vi "Server.vi"   [LabVIEW 2025]
uses:
  ServerGlobalVariables.vi
  ServerNetworkInterfaceGlobalVariables.vi
  <vilib>/Utility/miscctls.llb/LVMapReplaceAction.ctl
  bb7a831f-7d97-4d2b-be74-8b4a38f97bb1.vi
types:
  T1 = map{u32, cluster{"Name":string, "Team":u8, "Ready":bool, "Host":bool, "Alive":bool, "Color":u32, "Lands":set{cluster{"Row":u32, "Column":u32}}, "Army":u32}}
  T2 = enum16{"Init", "Lobby", "Game Init", "Game", "Game End"}
  T3 = enum16{"Wait Send Queue Ready", "Wait Receive Queue Ready", "Poll Read Queue", "Process Data"}
  T4 = cluster{"Data":string, "Address":u32, "Port":u16}
  T5 = enum16{"Wait Send Queue Ready", "Wait Receive Queue Ready", "Poll Read Queue", "Process Data", "Remove Land"}
  T6 = typedef "LVMapReplaceAction.ctl" = enum32{"Modify Entry only if found", "Add or Modify Entry", "Delete Entry"}
  T7 = cluster{"Name":string, "Team":u8, "Ready":bool, "Host":bool, "Alive":bool, "Color":u32, "Lands":set{cluster{"Row":u32, "Column":u32}}, "Army":u32}
  T8 = cluster{"string array[0]":string, "string array[1]":string, "string array[2]":string, "string array[3]":string}
  T9 = cluster{"Troops":u32, "Owner":i32, "Mountain":bool, "City":bool, "General":bool}[][]
  T10 = cluster{"Troops":u32, "Owner":i32, "Mountain":bool, "City":bool, "General":bool}
  T11 = cluster{"string array[0]":string, "string array[1]":string}
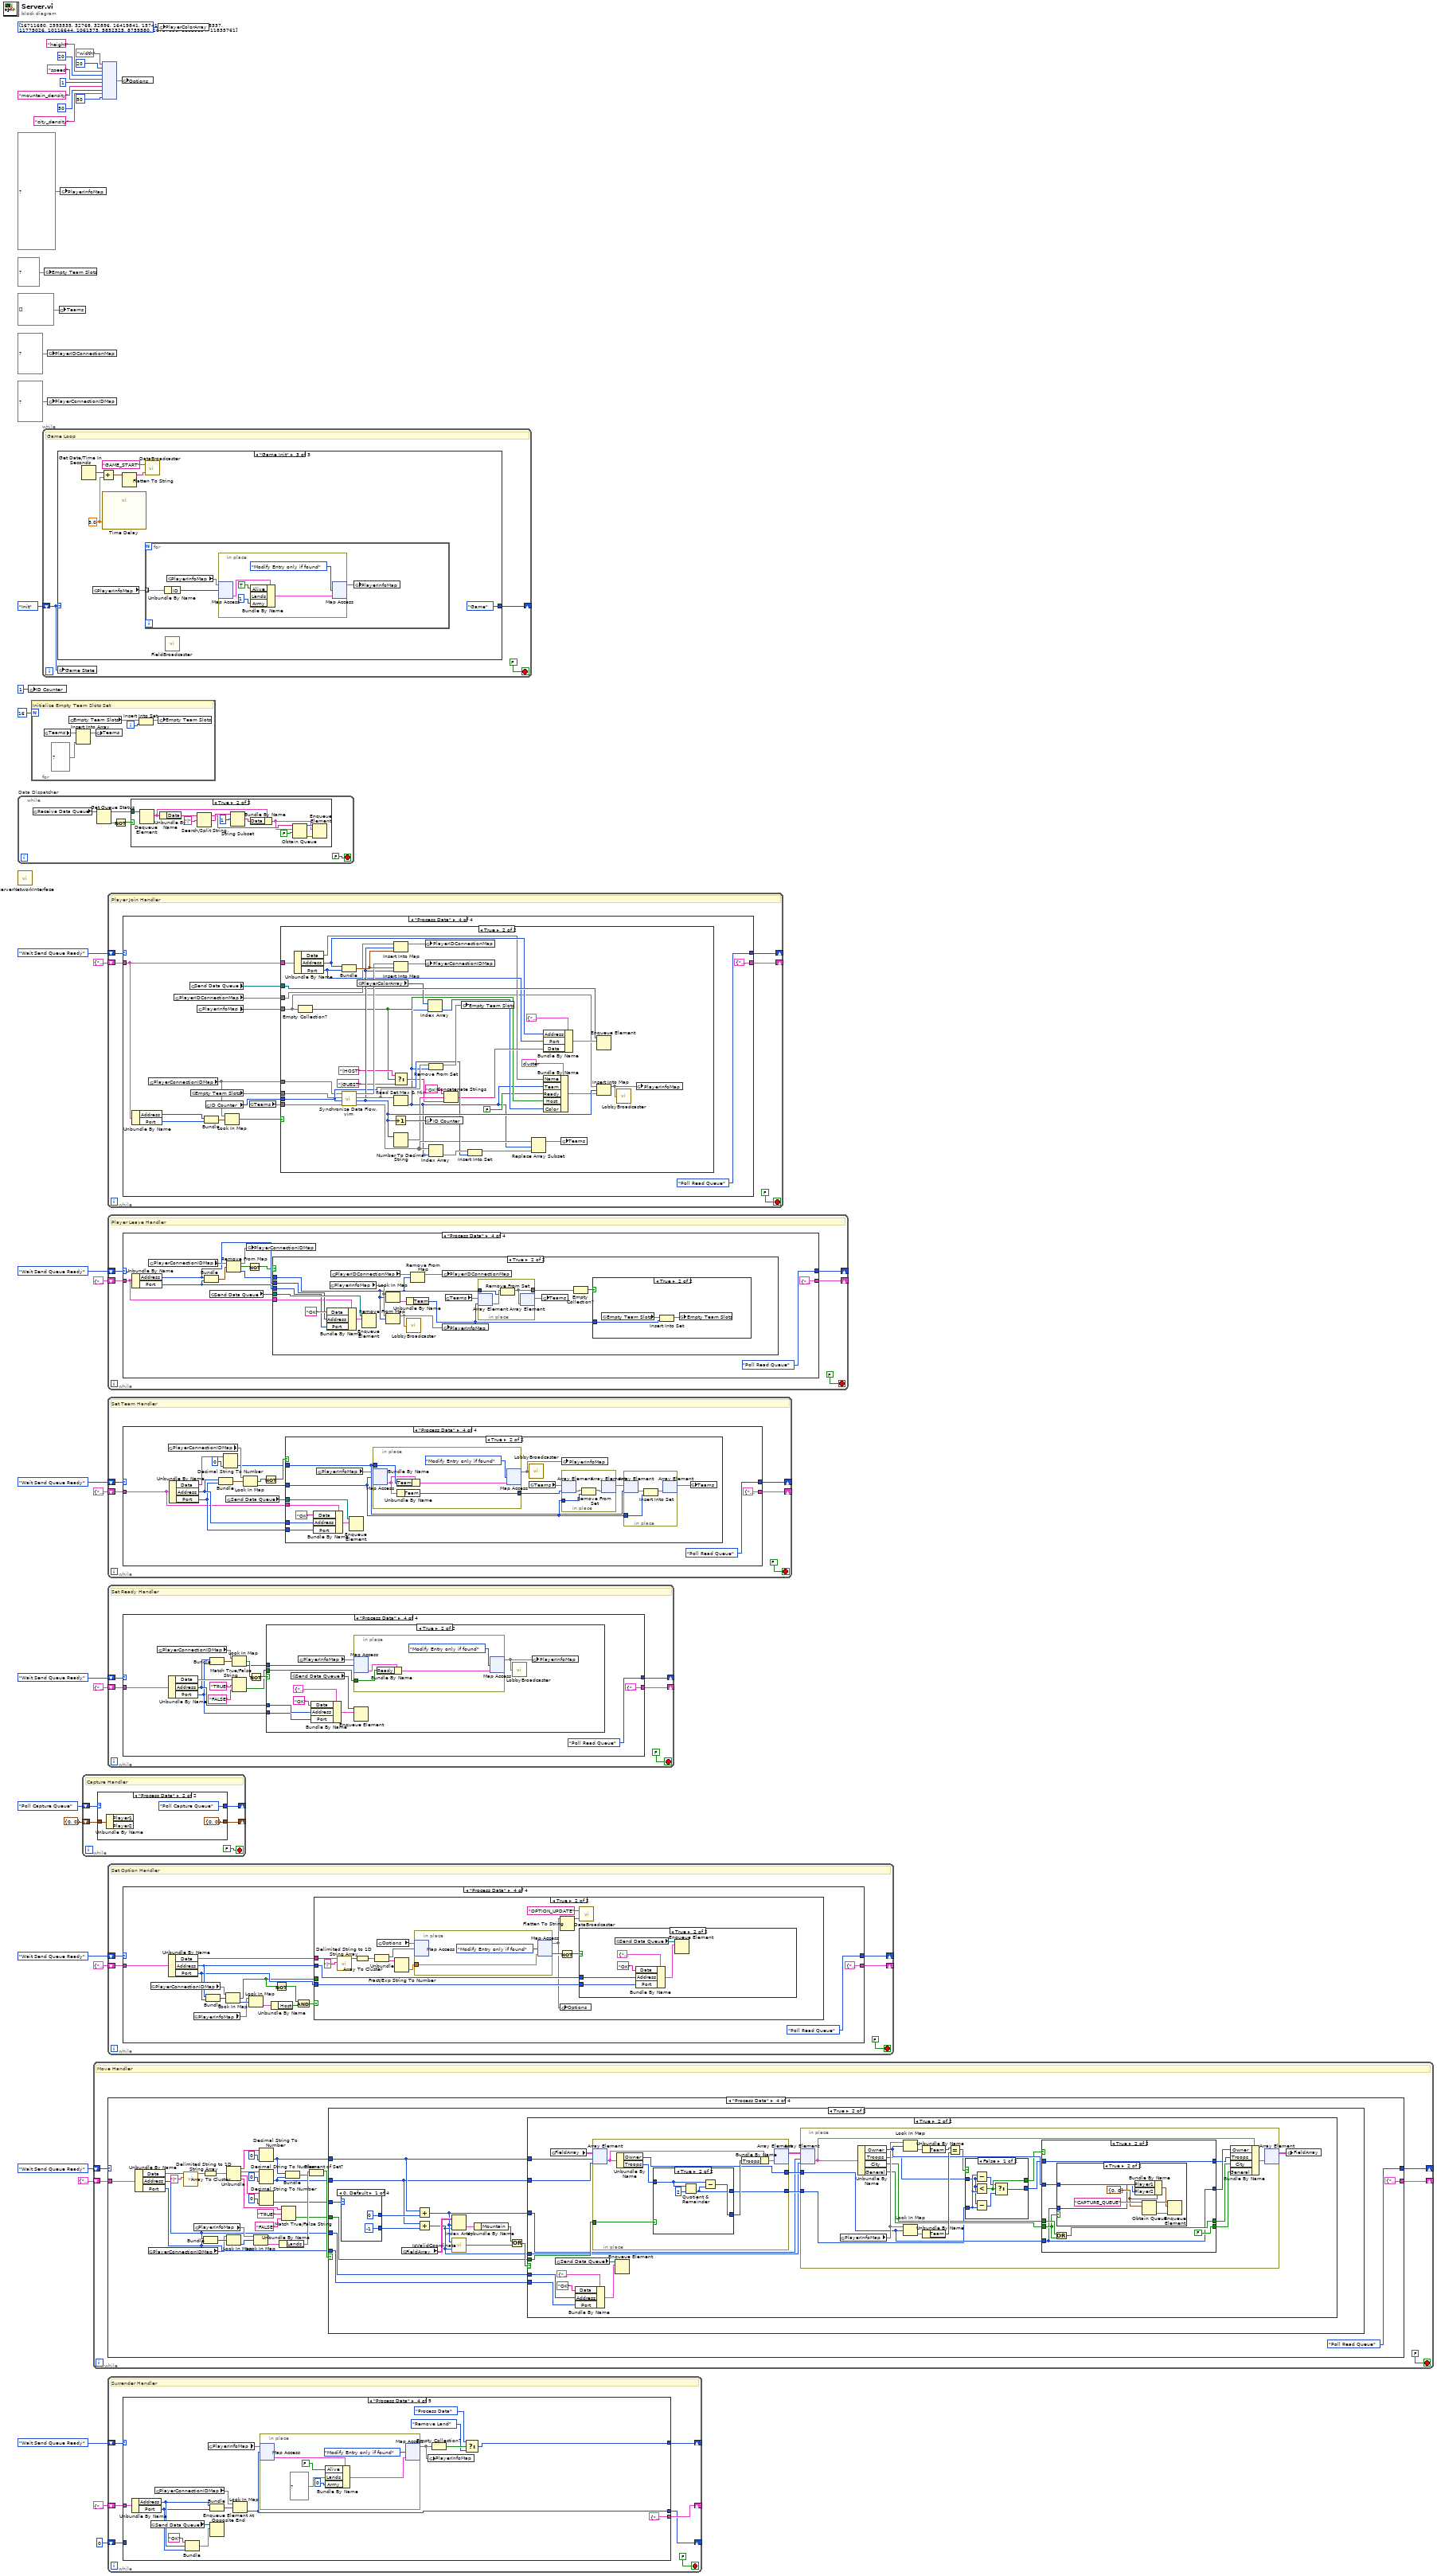
[diagram p0: block diagram]
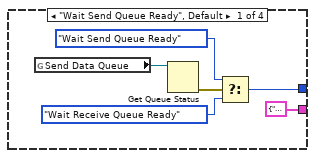
[diagram p2: hidden frame]
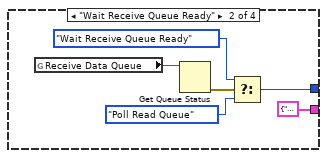
[diagram p3: hidden frame]
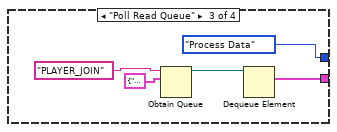
[diagram p4: hidden frame]
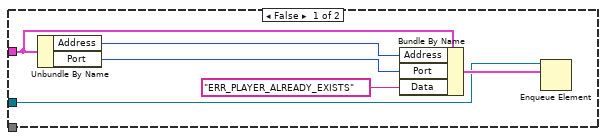
[diagram p5: hidden frame]
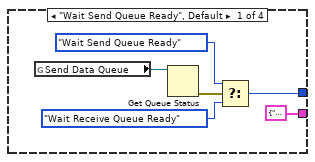
[diagram p6: hidden frame]
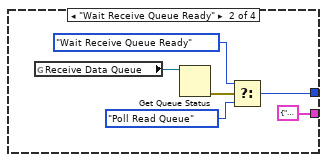
[diagram p7: hidden frame]
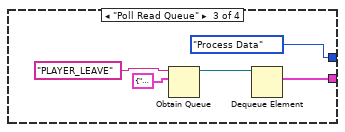
[diagram p8: hidden frame]
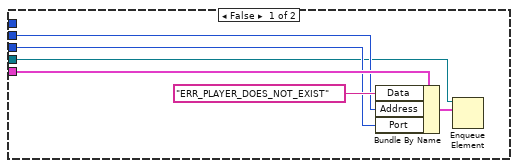
[diagram p9: hidden frame]
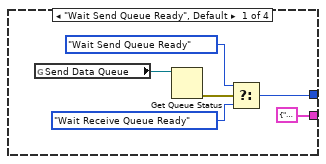
[diagram p11: hidden frame]
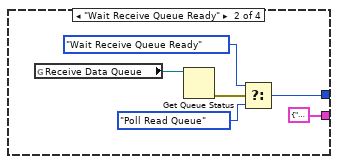
[diagram p12: hidden frame]
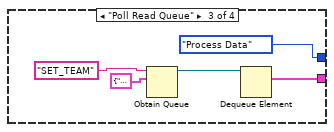
[diagram p13: hidden frame]
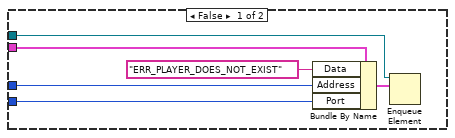
[diagram p14: hidden frame]
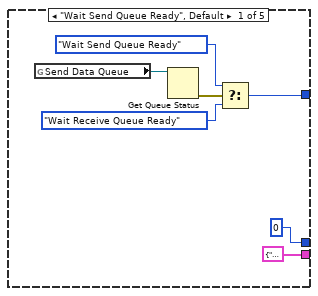
[diagram p15: hidden frame]
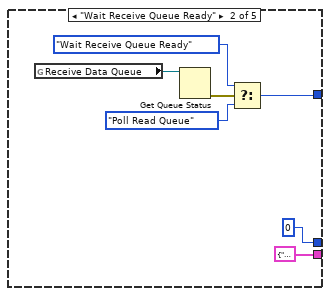
[diagram p16: hidden frame]
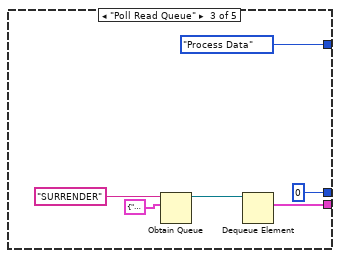
[diagram p17: hidden frame]
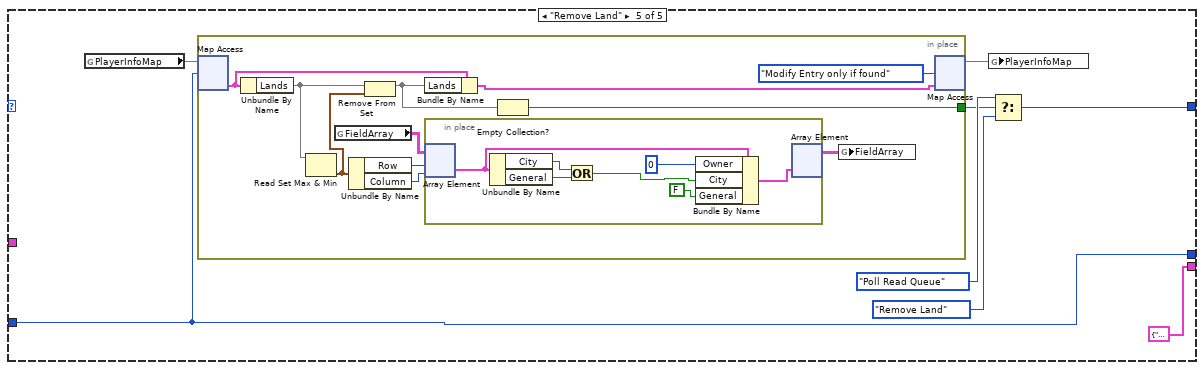
[diagram p18: hidden frame]
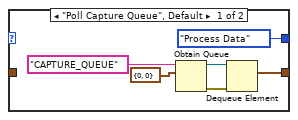
[diagram p19: hidden frame]
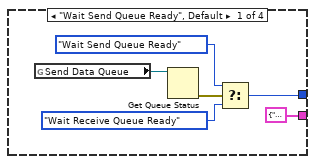
[diagram p20: hidden frame]
diagram:
  n1 = while "Data Dispatcher" {
    stop <- FALSE stop-if-true
    n2 = global read "ServerNetworkInterfaceGlobalVariables.vi" "Receive Data Queue"() -> (w41:refnum<queue>)
    n3 = Get Queue Status(queue=w41) -> (queue out=w38:refnum<queue>, error out=w40:errorcluster)  [unwired: 2 in, 6 out]
    n4 = Not(x=w40) -> (.not. x?=w39:bool)
    n5 = case shown="True" w39 {
      tunnel: w38 -> [_ w43]
      frame False {
      }
      frame True {
        n6 = Dequeue Element(queue=w43) -> (element=w50:T4)  [unwired: 2 in, 3 out]
        n7 = Unbundle By Name(w50) -> ("Data"=w54:string)
        n8 = Search/Split String(string=w54, search string/char (-)="|") -> (substring before match=w47:string, match + rest of string=w52:string)  [unwired: 1 in, 1 out]
        n9 = String Subset(string=w52, offset (0)=1) -> (substring=w49:string)  [unwired: 1 in]
        n10 = Bundle By Name(cluster=w50, "Data"=w49) -> (w44:T4)
        n11 = Obtain Queue(name (unnamed)=w47, element data type=w44, create if not found? (T)=FALSE) -> (queue out=w46:refnum<queue>, error out=w45:errorcluster)  [unwired: 2 in, 1 out]
        n12 = Enqueue Element(queue=w46, element=w44, error in (no error)=w45) -> ()  [unwired: 1 in, 3 out]
      }
    }
  }
  n13 = call "ServerNetworkInterface.vi"() -> ()  [unwired: 1 in]
  n14 = global write "ServerGlobalVariables.vi" "ID Counter"(u32 1 ("ID Counter")) -> ()
  n15 = for {
    N: 16 -> [_]
    i -> [w55]
    # "Initialize Empty Team Slots Set"
    n16 = global read "ServerGlobalVariables.vi" "Teams"() -> (w57:set{u32}[])
    n17 = global read "ServerGlobalVariables.vi" "Empty Team Slots"() -> (w60:set{u8})
    n18 = Insert Into Array(array=w57, new element=set{u32} {} ("new element/subarray")) -> (w58:set{u32}[])  [unwired: 1 in]
    n19 = global write "ServerGlobalVariables.vi" "Teams"(w58) -> ()
    n20 = Insert Into Set(10:w55, 11:w60) -> (3:w59:set{u8})  [unwired: 1 out]
    n21 = global write "ServerGlobalVariables.vi" "Empty Team Slots"(w59) -> ()
  }
  n22 = while {
    shift-right: [w61] -> _
    shift-left: T2."Init" -> [w62]
    stop <- FALSE stop-if-true
    # "Game Loop"
    n23 = case shown="\"Game Init\"" w62 {
      tunnel: [T2."Init" w65 T2."Game"] -> w61
      frame "Init", Default {
      }
      frame "Lobby" {
        n24 = global read "ServerGlobalVariables.vi" "PlayerInfoMap"() -> (w69:T1)
        n25 = Collection Size(1:w69) -> (0:w71:i32)
        n26 = for {
          N: w71 -> [_]
          shift-right: [w74] -> w68
          shift-left: TRUE -> [w72]
          tunnel: w69 -> [w75] mode=indexing
          n27 = Unbundle By Name(w75) -> ("PlayerInfo.Ready"=w73:bool)
          n28 = And(x=w73, y=w72) -> (x .and. y?=w74:bool)
        }
        n29 = Select(t=T2."Lobby", s=w68, f=T2."Game Init") -> (s? t:f=w65:T2)
      }
      frame "Game Init" {
        w77 = 3.0 ("y")
        n30 = Get Date/Time In Seconds() -> (seconds since 1Jan1904=w80:timestamp)
        n31 = global read "ServerGlobalVariables.vi" "PlayerInfoMap"() -> (w76:T1)
        n32 = Add(x=w80, y=w77) -> (x+y=w78:timestamp)
        n33 = call "Time Delay"("Delay Time (s)"=w77) -> ()  [unwired: 10 in, 1 out]
        n34 = Flatten To String(anything=w78) -> (data string=w79:string)  [unwired: 3 in, 2 out]
        n35 = call "DataBroadcaster.vi"("Data"=w79, "Action"="GAME_START") -> ()
        n36 = for {
          tunnel: w76 -> [w86] mode=indexing
          n37 = Unbundle By Name(w86) -> ("ID"=w84:u32)
          n38 = global read "ServerGlobalVariables.vi" "PlayerInfoMap"() -> (w85:T1)
          n39 = in-place {
            n40 = in-place-map #1(w85, w84) -> (w91:T7)  [unwired: 1 in, 1 out]
            n41 = Bundle By Name(cluster=w91, "Alive"=TRUE, "Army"=u32 1) -> (w88:T7)  [unwired: 1 in]
            n42 = in-place-map #1(w88, LVMapReplaceAction."Modify Entry only if found" ("action")) -> (w83:T1)  [unwired: 2 out]
          }
          n43 = global write "ServerGlobalVariables.vi" "PlayerInfoMap"(w83) -> ()
        }
        n44 = call "FieldBroadcaster.vi"() -> ()  [unwired: 12 in]
      }
    }
    n45 = global write "ServerGlobalVariables.vi" "Game State"(w62) -> ()
  }
  n46 = global write "ServerGlobalVariables.vi" "Empty Team Slots"(set{u8} {} ("Empty Team Slots")) -> ()
  n47 = global write "ServerGlobalVariables.vi" "PlayerIDConnectionMap"(map{u32, cluster{"Address":u32, "Port":u16}} {} ("PlayerIDConnectionMap")) -> ()
  n48 = global write "ServerGlobalVariables.vi" "PlayerConnectionIDMap"(map{cluster{"Address":u32, "Port":u16}, u32} {} ("PlayerConnectionIDMap")) -> ()
  n49 = global write "ServerGlobalVariables.vi" "Teams"(set{u32}[] [] ("Teams")) -> ()
  n50 = global write "ServerGlobalVariables.vi" "PlayerInfoMap"(T1 {} ("PlayerInfoMap")) -> ()
  n51 = while {
    shift-right: [w95] -> _
    shift-left: enum16{"Poll Capture Queue", "Process Data"}."Poll Capture Queue" -> [w96]
    shift-right: [w94] -> _
    shift-left: cluster{"Player1":u8, "Player2":u8} {"Player1"=0, "Player2"=0} -> [w93]
    stop <- FALSE stop-if-true
    # "Capture Handler"
    n52 = case shown="\"Process Data\"" w96 {
      tunnel: [enum16{"Poll Capture Queue", "Process Data"}."Process Data" enum16{"Poll Capture Queue", "Process Data"}."Poll Capture Queue"] -> w95
      tunnel: [w97 cluster{"Player1":u8, "Player2":u8} {"Player1"=0, "Player2"=0}] -> w94
      tunnel: w93 -> [_ w103]
      frame "Poll Capture Queue", Default {
        n53 = Obtain Queue(name (unnamed)="CAPTURE_QUEUE", element data type=cluster{"Player1":u8, "Player2":u8} {"Player1"=0, "Player2"=0}) -> (queue out=w99:refnum<queue>, error out=w98:errorcluster)  [unwired: 3 in, 1 out]
        n54 = Dequeue Element(queue=w99, error in (no error)=w98) -> (element=w97:cluster{"Player1":u8, "Player2":u8})  [unwired: 1 in, 3 out]
      }
      frame "Process Data" {
        n55 = Unbundle By Name(w103) -> ()  [unwired: 2 out]
      }
    }
  }
  n56 = while {
    shift-right: [w109] -> _
    shift-left: T3."Wait Send Queue Ready" -> [w106]
    shift-right: [w108] -> _
    shift-left: T4 {"Data"="", "Address"=0, "Port"=0} -> [w107]
    stop <- FALSE stop-if-true
    # "Move Handler"
    n57 = case shown="\"Process Data\"" w106 {
      tunnel: [w114 w118 T3."Process Data" T3."Poll Read Queue"] -> w109
      tunnel: [T4 {"Data"="", "Address"=0, "Port"=0} T4 {"Data"="", "Address"=0, "Port"=0} w124 T4 {"Data"="", "Address"=0, "Port"=0}] -> w108
      tunnel: w107 -> [_ _ _ w137]
      frame "Wait Send Queue Ready", Default {
        n58 = global read "ServerNetworkInterfaceGlobalVariables.vi" "Send Data Queue"() -> (w116:refnum<queue>)
        n59 = Get Queue Status(queue=w116) -> (error out=w115:errorcluster)  [unwired: 2 in, 7 out]
        n60 = Select(t=T3."Wait Send Queue Ready", s=w115, f=T3."Wait Receive Queue Ready") -> (s? t:f=w114:T3)
      }
      frame "Wait Receive Queue Ready" {
        n61 = global read "ServerNetworkInterfaceGlobalVariables.vi" "Receive Data Queue"() -> (w121:refnum<queue>)
        n62 = Get Queue Status(queue=w121) -> (error out=w122:errorcluster)  [unwired: 2 in, 7 out]
        n63 = Select(t=T3."Wait Receive Queue Ready", s=w122, f=T3."Poll Read Queue") -> (s? t:f=w118:T3)
      }
      frame "Poll Read Queue" {
        n64 = Obtain Queue(name (unnamed)="MOVE", element data type=T4 {"Data"="", "Address"=0, "Port"=0}) -> (queue out=w125:refnum<queue>)  [unwired: 3 in, 2 out]
        n65 = Dequeue Element(queue=w125) -> (element=w124:T4)  [unwired: 2 in, 3 out]
      }
      frame "Process Data" {
        n66 = Unbundle By Name(w137) -> ("Data"=w148:string, "Address"=w132:u32, "Port"=w133:u16)
        n67 = global read "ServerGlobalVariables.vi" "PlayerConnectionIDMap"() -> (w154:map{cluster{"Address":u32, "Port":u16}, u32})
        n68 = call <vilib>:"Delimited String to 1D String Array.vi"("delimiter"="|", "delimited string"=w148) -> ("string array"=w149:string[])  [unwired: 9 in]
        n69 = global read "ServerGlobalVariables.vi" "PlayerInfoMap"() -> (w152:T1)
        n70 = Array To Cluster(array=w149) -> (cluster=w142:T8)
        n71 = Bundle("Address"=w132, "Port"=w133) -> (w155:cluster{"Address":u32, "Port":u16})  [unwired: 1 in]
        n72 = Unbundle(w142) -> ("string array[0]"=w138:string, "string array[1]"=w139:string, "string array[2]"=w140:string, "string array[3]"=w141:string)
        n73 = Look In Map(map=w154, key=w155) -> (value=w153:u32)  [unwired: 1 in, 1 out]
        n74 = Look In Map(map=w152, key=w153) -> (value=w151:T7)  [unwired: 1 in, 1 out]
        n75 = Decimal String To Number(string=w138, default (0L)=u32 0 ("default (0 I32)")) -> (number=w130:u32)  [unwired: 1 in, 1 out]
        n76 = Decimal String To Number(string=w139, default (0L)=u32 0 ("default (0 I32)")) -> (number=w129:u32)  [unwired: 1 in, 1 out]
        n77 = Decimal String To Number(string=w140, default (0L)=u32 0 ("default (0 I32)")) -> (number=w131:u32)  [unwired: 1 in, 1 out]
        n78 = Unbundle By Name(w151) -> ("Lands"=w136:set{cluster{"Row":u32, "Column":u32}})
        n79 = Match True/False String(2:"FALSE" ("false string"), 3:"TRUE" ("true string"), 4:w141) -> (0:w128:bool)  [unwired: 1 out]
        n80 = Bundle(w130, w129) -> (w135:cluster{u32, u32})  [unwired: 1 in]
        n81 = Element of Set?(10:w135, 11:w136) -> (3:w134:bool)
        n82 = case shown="True" w134 {
          tunnel: w133 -> [w159 w174]
          tunnel: w132 -> [w158 w175]
          tunnel: w131 -> [_ w178]
          tunnel: w130 -> [_ w167]
          tunnel: w129 -> [_ w166]
          tunnel: w128 -> [_ w168]
          frame False {
            n83 = global read "ServerNetworkInterfaceGlobalVariables.vi" "Send Data Queue"() -> (w160:refnum<queue>)
            n84 = Bundle By Name(cluster=T4 {"Data"="", "Address"=0, "Port"=0}, "Data"="ERR_NOT_OWN_LAND", "Address"=w158, "Port"=w159) -> (w162:T4)
            n85 = Enqueue Element(queue=w160, element=w162) -> ()  [unwired: 2 in, 3 out]
          }
          frame True {
            n86 = case shown="0, Default" w178 {
              tunnel: [-1 0 1 0] -> w177
              tunnel: [0 1 0 -1] -> w176
              frame 0, Default {
              }
              frame 1 {
              }
              frame 2 {
              }
              frame 3 {
              }
            }
            n87 = global read "ServerGlobalVariables.vi" "FieldArray"() -> (w173:T9)
            n88 = Add(x=w167, y=w176) -> (x+y=w165:u32)
            n89 = Add(x=w166, y=w177) -> (x+y=w164:u32)
            n90 = Index Array(array=w173, index (row)=w165, index (col)=w164) -> (element=w169:T10)
            n91 = call "IsValidCoordinate.vi"("Column"=w164, "Row"=w165) -> ("Valid"=w171:bool)
            n92 = Unbundle By Name(w169) -> ("Mountain"=w172:bool)
            n93 = Or(x=w172, y=w171) -> (x .or. y?=w170:bool)
            n94 = case shown="True" w170 {
              tunnel: w175 -> [w180 w192]
              tunnel: w174 -> [w179 w191]
              tunnel: w168 -> [_ w197]
              tunnel: w167 -> [_ w200]
              tunnel: w166 -> [_ w199]
              tunnel: w165 -> [_ w187]
              tunnel: w164 -> [_ w186]
              frame False {
                n95 = global read "ServerNetworkInterfaceGlobalVariables.vi" "Send Data Queue"() -> (w181:refnum<queue>)
                n96 = Bundle By Name(cluster=T4 {"Data"="", "Address"=0, "Port"=0}, "Data"="ERR_INVALID_MOVE", "Address"=w180, "Port"=w179) -> (w183:T4)
                n97 = Enqueue Element(queue=w181, element=w183) -> ()  [unwired: 2 in, 3 out]
              }
              frame True {
                n98 = global read "ServerGlobalVariables.vi" "FieldArray"() -> (w198:T9)
                n99 = global read "ServerNetworkInterfaceGlobalVariables.vi" "Send Data Queue"() -> (w193:refnum<queue>)
                n100 = Bundle By Name(cluster=T4 {"Data"="", "Address"=0, "Port"=0}, "Data"="OK", "Address"=w192, "Port"=w191) -> (w195:T4)
                n101 = in-place {
                  in-place-border: w197 -> [w251]
                  in-place-border: [w253] -> w190
                  in-place-border: [w252] -> w189
                  n102 = in-place-array #2(w198, w200, w199) -> (w256:T10)
                  n103 = Unbundle By Name(w256) -> ("Owner"=w253:i32, "Troops"=w257:u32)
                  n104 = case shown="True" w251 {
                    tunnel: [w264 w269] -> w254
                    tunnel: [w265 w267] -> w252
                    tunnel: w257 -> [w261 w266]
                    frame False {
                      n105 = Decrement(x=w261) -> (x-1=w262:u32)
                      n106 = Greater Than 0?(x=w261) -> (x > 0?=w263:bool)
                      n107 = Select(t=w262, s=w263, f=u32 0) -> (s? t:f=w265:u32)
                      n108 = Select(t=u32 1, s=w263, f=u32 0) -> (s? t:f=w264:u32)
                    }
                    frame True {
                      n109 = Quotient & Remainder(x=w266, y=u32 2) -> (floor(x/y)=w267:u32)  [unwired: 1 out]
                      n110 = Subtract(x=w266, y=w267) -> (x-y=w269:u32)
                    }
                  }
                  n111 = Bundle By Name(cluster=w256, "Troops"=w254) -> (w255:T10)
                  n112 = in-place-array #2(w255) -> (w188:T9)  [unwired: 2 out]
                }
                n113 = Enqueue Element(queue=w193, element=w195) -> ()  [unwired: 2 in, 3 out]
                n114 = in-place {
                  in-place-border: w190 -> [w204]
                  in-place-border: w189 -> [w203]
                  n115 = in-place-array #3(w188, w187, w186) -> (w202:T10)
                  n116 = global read "ServerGlobalVariables.vi" "PlayerInfoMap"() -> (w215:T1)
                  n117 = Unbundle By Name(w202) -> ("Owner"=w216:i32, "Troops"=w206:u32, "City"=w208:bool, "General"=w212:bool)
                  n118 = Look In Map(map=w215, key=w216) -> (value=w218:T7)  [unwired: 1 in, 1 out]
                  n119 = Look In Map(map=w215, key=w204) -> (value=w217:T7)  [unwired: 1 in, 1 out]
                  n120 = Unbundle By Name(w218) -> ("Team"=w219:u8)
                  n121 = Unbundle By Name(w217) -> ("Team"=w220:u8)
                  n122 = Equal?(x=w219, y=w220) -> (x = y?=w205:bool)
                  n123 = case shown="False" w205 {
                    tunnel: w206 -> [w242 w250]
                    tunnel: w203 -> [w243 w249]
                    tunnel: [w246 w248] -> w209
                    tunnel: [w244 FALSE] -> w207
                    frame False {
                      n124 = Subtract(x=w243, y=w242) -> (x-y=w241:u32)
                      n125 = Less?(x=w242, y=w243) -> (x < y?=w244:bool)
                      n126 = Subtract(x=w242, y=w243) -> (x-y=w245:u32)
                      n127 = Select(t=w241, s=w244, f=w245) -> (s? t:f=w246:u32)
                    }
                    frame True {
                      n128 = Add(x=w250, y=w249) -> (x+y=w248:u32)
                    }
                  }
                  n129 = case shown="True" w207 {
                    tunnel: w208 -> [w225 w232]
                    tunnel: w209 -> [w226 w233]
                    tunnel: [w226 w233] -> w210
                    tunnel: w204 -> [w222 w228]
                    tunnel: w216 -> [w224 w227]
                    tunnel: [w221 w228] -> w211
                    tunnel: w212 -> [w223 w229]
                    tunnel: [w225 w231] -> w213
                    tunnel: [w223 FALSE ("General")] -> w214
                    frame False {
                      n130 = Select(t=w224, s=w223, f=w222) -> (s? t:f=w221:i32)
                    }
                    frame True {
                      n131 = Or(x=w232, y=w229) -> (x .or. y?=w231:bool)
                      n132 = case shown="True" w229 {
                        tunnel: w228 -> [_ w236]
                        tunnel: w227 -> [_ w235]
                        frame False {
                        }
                        frame True {
                          w237 = cluster{"Player1":u8, "Player2":u8} {"Player1"=0, "Player2"=0}
                          n133 = Bundle By Name(cluster=w237, "Player1"=w236, "Player2"=w235) -> (w234:cluster{"Player1":u8, "Player2":u8})
                          n134 = Obtain Queue(name (unnamed)="CAPTURE_QUEUE", element data type=w237) -> (queue out=w239:refnum<queue>, error out=w238:errorcluster)  [unwired: 3 in, 1 out]
                          n135 = Enqueue Element(queue=w239, element=w234, error in (no error)=w238) -> ()  [unwired: 1 in, 3 out]
                        }
                      }
                    }
                  }
                  n136 = Bundle By Name(cluster=w202, "Owner"=w211, "Troops"=w210, "City"=w213, "General"=w214) -> (w201:T10)
                  n137 = in-place-array #3(w201) -> (w185:T9)  [unwired: 2 out]
                }
                n138 = global write "ServerGlobalVariables.vi" "FieldArray"(w185) -> ()
              }
            }
          }
        }
      }
    }
  }
  n139 = node("width" ("key"), u32 20 ("value"), "height" ("key"), u32 20 ("value"), "speed" ("key"), u32 1 ("value"), "mountain_density" ("key"), u32 50 ("value"), "city_density" ("key"), u32 50 ("value")) -> (w21:map{string, u32})
  n140 = while {
    shift-right: [w281] -> _
    shift-left: T3."Wait Send Queue Ready" -> [w278]
    shift-right: [w280] -> _
    shift-left: T4 {"Data"="", "Address"=0, "Port"=0} -> [w279]
    stop <- FALSE stop-if-true
    # "Player Join Handler"
    n141 = case shown="\"Process Data\"" w278 {
      tunnel: [w286 w290 T3."Process Data" T3."Poll Read Queue"] -> w281
      tunnel: [T4 {"Data"="", "Address"=0, "Port"=0} T4 {"Data"="", "Address"=0, "Port"=0} w296 T4 {"Data"="", "Address"=0, "Port"=0}] -> w280
      tunnel: w279 -> [_ _ _ w300]
      frame "Wait Send Queue Ready", Default {
        n142 = global read "ServerNetworkInterfaceGlobalVariables.vi" "Send Data Queue"() -> (w288:refnum<queue>)
        n143 = Get Queue Status(queue=w288) -> (error out=w287:errorcluster)  [unwired: 2 in, 7 out]
        n144 = Select(t=T3."Wait Send Queue Ready", s=w287, f=T3."Wait Receive Queue Ready") -> (s? t:f=w286:T3)
      }
      frame "Wait Receive Queue Ready" {
        n145 = global read "ServerNetworkInterfaceGlobalVariables.vi" "Receive Data Queue"() -> (w293:refnum<queue>)
        n146 = Get Queue Status(queue=w293) -> (error out=w294:errorcluster)  [unwired: 2 in, 7 out]
        n147 = Select(t=T3."Wait Receive Queue Ready", s=w294, f=T3."Poll Read Queue") -> (s? t:f=w290:T3)
      }
      frame "Poll Read Queue" {
        n148 = Obtain Queue(name (unnamed)="PLAYER_JOIN", element data type=T4 {"Data"="", "Address"=0, "Port"=0}) -> (queue out=w297:refnum<queue>)  [unwired: 3 in, 2 out]
        n149 = Dequeue Element(queue=w297) -> (element=w296:T4)  [unwired: 2 in, 3 out]
      }
      frame "Process Data" {
        n150 = Unbundle By Name(w300) -> ("Address"=w303:u32, "Port"=w304:u16)
        n151 = global read "ServerGlobalVariables.vi" "PlayerConnectionIDMap"() -> (w306:map{cluster{"Address":u32, "Port":u16}, u32})
        n152 = global read "ServerGlobalVariables.vi" "PlayerIDConnectionMap"() -> (w310:map{u32, cluster{"Address":u32, "Port":u16}})
        n153 = global read "ServerNetworkInterfaceGlobalVariables.vi" "Send Data Queue"() -> (w301:refnum<queue>)
        n154 = global read "ServerGlobalVariables.vi" "Empty Team Slots"() -> (w309:set{u8})
        n155 = global read "ServerGlobalVariables.vi" "PlayerInfoMap"() -> (w311:T1)
        n156 = Bundle("Address"=w303, "Port"=w304) -> (w302:cluster{"Address":u32, "Port":u16})  [unwired: 1 in]
        n157 = global read "ServerGlobalVariables.vi" "ID Counter"() -> (w307:u32)
        n158 = Look In Map(map=w306, key=w302) -> (key not found?=w305:bool)  [unwired: 1 in, 1 out]
        n159 = global read "ServerGlobalVariables.vi" "Teams"() -> (w308:set{u32}[])
        n160 = case shown="True" w305 {
          tunnel: w311 -> [_ w322]
          tunnel: w310 -> [_ w353]
          tunnel: w300 -> [w315 w352]
          tunnel: w309 -> [_ w350]
          tunnel: w301 -> [w318 w347]
          tunnel: w308 -> [_ w346]
          tunnel: w307 -> [_ w344]
          tunnel: w306 -> [_ w335]
          frame False {
            n161 = Unbundle By Name(w315) -> ("Address"=w317:u32, "Port"=w316:u16)
            n162 = Bundle By Name(cluster=w315, "Address"=w317, "Port"=w316, "Data"="ERR_PLAYER_ALREADY_EXISTS") -> (w319:T4)
            n163 = Enqueue Element(queue=w318, element=w319) -> ()  [unwired: 2 in, 3 out]
          }
          frame True {
            n164 = Unbundle By Name(w352) -> ("Data"=w323:string, "Address"=w339:u32, "Port"=w338:u16)
            n165 = Empty Collection?(1:w322) -> (0:w326:bool)
            n166 = Bundle("Address"=w339, "Port"=w338) -> (w354:cluster{"Address":u32, "Port":u16})  [unwired: 1 in]
            n167 = call "Synchronize Data Flow.vim"("input 4"=w346, "input 3"=w344, "input 2"=w350, "input 1"=w335) -> ("output 4"=w343:set{u32}[], "output 3"=w348:u32, "output 2"=w349:set{u8}, "output 1"=w351:map{cluster{"Address":u32, "Port":u16}, u32})
            n168 = global read "ServerGlobalVariables.vi" "PlayerColorArray"() -> (w329:u32[])
            n169 = Increment(x=w348) -> (x+1=w358:u32)
            n170 = Insert Into Map(map in=w353, key=w348, value=w354) -> (map out=w355:map{u32, cluster{"Address":u32, "Port":u16}})  [unwired: 2 out]
            n171 = Insert Into Map(map in=w351, key=w354, value=w348) -> (map out=w357:map{cluster{"Address":u32, "Port":u16}, u32})  [unwired: 2 out]
            n172 = Select(t="|HOST", s=w326, f="|GUEST") -> (s? t:f=w330:string)
            n173 = Read Set Max & Min(11:w349) -> (1:w324:u8)  [unwired: 1 out]
            n174 = Number To Decimal String(number=w348) -> (decimal integer string=w337:string)  [unwired: 1 in]
            n175 = global write "ServerGlobalVariables.vi" "PlayerIDConnectionMap"(w355) -> ()
            n176 = global write "ServerGlobalVariables.vi" "PlayerConnectionIDMap"(w357) -> ()
            n177 = global write "ServerGlobalVariables.vi" "ID Counter"(w358) -> ()
            n178 = Index Array(array=w329, index=w324) -> (element=w327:u32)
            n179 = Index Array(array=w343, index=w324) -> (element=w345:set{u32})
            n180 = Remove From Set(10:w324, 11:w349) -> (3:w356:set{u8})  [unwired: 1 out]
            n181 = Concatenate Strings("OK|" ("string"), w337, w330) -> (w334:string)
            n182 = global write "ServerGlobalVariables.vi" "Empty Team Slots"(w356) -> ()
            n183 = Insert Into Set(10:w344, 11:w345) -> (3:w342:set{u32})  [unwired: 1 out]
            n184 = Replace Array Subset(array=w343, new element=w342, index=w324) -> (w341:set{u32}[])
            n185 = Bundle By Name(cluster=T4 {"Data"="", "Address"=0, "Port"=0}, "Address"=w339, "Port"=w338, "Data"=w334) -> (w336:T4)
            n186 = Bundle By Name(cluster=T7 {"Name"="", "Team"=0, "Ready"=FALSE, "Host"=FALSE, "Alive"=FALSE, "Color"=0, "Lands"={}, "Army"=0} ("PlayerInfo"), "Name"=w323, "Team"=w324, "Ready"=FALSE, "Host"=w326, "Color"=w327) -> (w321:T7)
            n187 = global write "ServerGlobalVariables.vi" "Teams"(w341) -> ()
            n188 = Enqueue Element(queue=w347, element=w336) -> ()  [unwired: 2 in, 3 out]
            n189 = Insert Into Map(map in=w322, key=w348, value=w321) -> (map out=w320:T1)  [unwired: 2 out]
            n190 = call "LobbyBroadcaster.vi"("PlayerInfoMap"=w320) -> ()
            n191 = global write "ServerGlobalVariables.vi" "PlayerInfoMap"(w320) -> ()
          }
        }
      }
    }
  }
  n192 = while {
    shift-right: [w362] -> _
    shift-left: T3."Wait Send Queue Ready" -> [w359]
    shift-right: [w361] -> _
    shift-left: T4 {"Data"="", "Address"=0, "Port"=0} -> [w360]
    stop <- FALSE stop-if-true
    # "Player Leave Handler"
    n193 = case shown="\"Process Data\"" w359 {
      tunnel: [w367 w371 T3."Process Data" T3."Poll Read Queue"] -> w362
      tunnel: [T4 {"Data"="", "Address"=0, "Port"=0} T4 {"Data"="", "Address"=0, "Port"=0} w377 T4 {"Data"="", "Address"=0, "Port"=0}] -> w361
      tunnel: w360 -> [_ _ _ w381]
      frame "Wait Send Queue Ready", Default {
        n194 = global read "ServerNetworkInterfaceGlobalVariables.vi" "Send Data Queue"() -> (w369:refnum<queue>)
        n195 = Get Queue Status(queue=w369) -> (error out=w368:errorcluster)  [unwired: 2 in, 7 out]
        n196 = Select(t=T3."Wait Send Queue Ready", s=w368, f=T3."Wait Receive Queue Ready") -> (s? t:f=w367:T3)
      }
      frame "Wait Receive Queue Ready" {
        n197 = global read "ServerNetworkInterfaceGlobalVariables.vi" "Receive Data Queue"() -> (w374:refnum<queue>)
        n198 = Get Queue Status(queue=w374) -> (error out=w375:errorcluster)  [unwired: 2 in, 7 out]
        n199 = Select(t=T3."Wait Receive Queue Ready", s=w375, f=T3."Poll Read Queue") -> (s? t:f=w371:T3)
      }
      frame "Poll Read Queue" {
        n200 = Obtain Queue(name (unnamed)="PLAYER_LEAVE", element data type=T4 {"Data"="", "Address"=0, "Port"=0}) -> (queue out=w378:refnum<queue>)  [unwired: 3 in, 2 out]
        n201 = Dequeue Element(queue=w378) -> (element=w377:T4)  [unwired: 2 in, 3 out]
      }
      frame "Process Data" {
        n202 = Unbundle By Name(w381) -> ("Address"=w388:u32, "Port"=w387:u16)
        n203 = global read "ServerGlobalVariables.vi" "PlayerConnectionIDMap"() -> (w389:map{cluster{"Address":u32, "Port":u16}, u32})
        n204 = Bundle("Address"=w388, "Port"=w387) -> (w390:cluster{"Address":u32, "Port":u16})  [unwired: 1 in]
        n205 = global read "ServerNetworkInterfaceGlobalVariables.vi" "Send Data Queue"() -> (w382:refnum<queue>)
        n206 = Remove From Map(10:w390, 11:w389) -> (1:w386:u32, 2:w384:bool, 3:w383:map{cluster{"Address":u32, "Port":u16}, u32})
        n207 = global write "ServerGlobalVariables.vi" "PlayerConnectionIDMap"(w383) -> ()
        n208 = Not(x=w384) -> (.not. x?=w385:bool)
        n209 = case shown="True" w385 {
          tunnel: w382 -> [w393 w413]
          tunnel: w388 -> [w395 w411]
          tunnel: w387 -> [w394 w410]
          tunnel: w386 -> [_ w402]
          tunnel: w381 -> [w396 w408]
          frame False {
            n210 = Bundle By Name(cluster=w396, "Data"="ERR_PLAYER_DOES_NOT_EXIST", "Address"=w395, "Port"=w394) -> (w397:T4)
            n211 = Enqueue Element(queue=w393, element=w397) -> ()  [unwired: 2 in, 3 out]
          }
          frame True {
            n212 = Bundle By Name(cluster=w408, "Data"="OK", "Address"=w411, "Port"=w410) -> (w409:T4)
            n213 = global read "ServerGlobalVariables.vi" "PlayerInfoMap"() -> (w403:T1)
            n214 = global read "ServerGlobalVariables.vi" "PlayerIDConnectionMap"() -> (w400:map{u32, cluster{"Address":u32, "Port":u16}})
            n215 = Enqueue Element(queue=w413, element=w409) -> ()  [unwired: 2 in, 3 out]
            n216 = Look In Map(map=w403, key=w402) -> (value=w415:T7)  [unwired: 1 in, 1 out]
            n217 = Remove From Map(10:w402, 11:w403) -> (3:w399:T1)  [unwired: 2 out]
            n218 = Unbundle By Name(w415) -> ("Team"=w407:u8)
            n219 = call "LobbyBroadcaster.vi"("PlayerInfoMap"=w399) -> ()
            n220 = Remove From Map(10:w402, 11:w400) -> (3:w401:map{u32, cluster{"Address":u32, "Port":u16}})  [unwired: 2 out]
            n221 = global write "ServerGlobalVariables.vi" "PlayerIDConnectionMap"(w401) -> ()
            n222 = global write "ServerGlobalVariables.vi" "PlayerInfoMap"(w399) -> ()
            n223 = global read "ServerGlobalVariables.vi" "Teams"() -> (w404:set{u32}[])
            n224 = in-place {
              in-place-border: w402 -> [w417]
              in-place-border: [w416] -> w406
              n225 = in-place-array #4(w404, w407) -> (w418:set{u32})
              n226 = Remove From Set(10:w417, 11:w418) -> (3:w416:set{u32})  [unwired: 1 out]
              n227 = in-place-array #4(w416) -> (w405:set{u32}[])  [unwired: 1 out]
            }
            n228 = global write "ServerGlobalVariables.vi" "Teams"(w405) -> ()
            n229 = Empty Collection?(1:w406) -> (0:w414:bool)
            n230 = case shown="True" w414 {
              tunnel: w407 -> [_ w421]
              frame False {
              }
              frame True {
                n231 = global read "ServerGlobalVariables.vi" "Empty Team Slots"() -> (w419:set{u8})
                n232 = Insert Into Set(10:w421, 11:w419) -> (3:w420:set{u8})  [unwired: 1 out]
                n233 = global write "ServerGlobalVariables.vi" "Empty Team Slots"(w420) -> ()
              }
            }
          }
        }
      }
    }
  }
  n234 = while {
    shift-right: [w425] -> _
    shift-left: T3."Wait Send Queue Ready" -> [w422]
    shift-right: [w424] -> _
    shift-left: T4 {"Data"="", "Address"=0, "Port"=0} -> [w423]
    stop <- FALSE stop-if-true
    # "Set Team Handler"
    n235 = case shown="\"Process Data\"" w422 {
      tunnel: [w430 w434 T3."Process Data" T3."Poll Read Queue"] -> w425
      tunnel: [T4 {"Data"="", "Address"=0, "Port"=0} T4 {"Data"="", "Address"=0, "Port"=0} w440 T4 {"Data"="", "Address"=0, "Port"=0}] -> w424
      tunnel: w423 -> [_ _ _ w444]
      frame "Wait Send Queue Ready", Default {
        n236 = global read "ServerNetworkInterfaceGlobalVariables.vi" "Send Data Queue"() -> (w432:refnum<queue>)
        n237 = Get Queue Status(queue=w432) -> (error out=w431:errorcluster)  [unwired: 2 in, 7 out]
        n238 = Select(t=T3."Wait Send Queue Ready", s=w431, f=T3."Wait Receive Queue Ready") -> (s? t:f=w430:T3)
      }
      frame "Wait Receive Queue Ready" {
        n239 = global read "ServerNetworkInterfaceGlobalVariables.vi" "Receive Data Queue"() -> (w437:refnum<queue>)
        n240 = Get Queue Status(queue=w437) -> (error out=w438:errorcluster)  [unwired: 2 in, 7 out]
        n241 = Select(t=T3."Wait Receive Queue Ready", s=w438, f=T3."Poll Read Queue") -> (s? t:f=w434:T3)
      }
      frame "Poll Read Queue" {
        n242 = Obtain Queue(name (unnamed)="SET_TEAM", element data type=T4 {"Data"="", "Address"=0, "Port"=0}) -> (queue out=w441:refnum<queue>)  [unwired: 3 in, 2 out]
        n243 = Dequeue Element(queue=w441) -> (element=w440:T4)  [unwired: 2 in, 3 out]
      }
      frame "Process Data" {
        n244 = global read "ServerGlobalVariables.vi" "PlayerConnectionIDMap"() -> (w455:map{cluster{"Address":u32, "Port":u16}, u32})
        n245 = Unbundle By Name(w444) -> ("Data"=w447:string, "Address"=w450:u32, "Port"=w449:u16)
        n246 = Bundle("Address"=w450, "Port"=w449) -> (w454:cluster{"Address":u32, "Port":u16})  [unwired: 1 in]
        n247 = Decimal String To Number(string=w447, default (0L)=u8 0 ("default (0 I32)")) -> (number=w446:u8)  [unwired: 1 in, 1 out]
        n248 = global read "ServerNetworkInterfaceGlobalVariables.vi" "Send Data Queue"() -> (w445:refnum<queue>)
        n249 = Look In Map(map=w455, key=w454) -> (key not found?=w452:bool, value=w451:u32)  [unwired: 1 in]
        n250 = Not(x=w452) -> (.not. x?=w453:bool)
        n251 = case shown="True" w453 {
          tunnel: w451 -> [_ w468]
          tunnel: w450 -> [w461 w473]
          tunnel: w449 -> [w460 w472]
          tunnel: w444 -> [w459 w474]
          tunnel: w445 -> [w458 w475]
          tunnel: w446 -> [_ w469]
          frame False {
            n252 = Bundle By Name(cluster=w459, "Data"="ERR_PLAYER_DOES_NOT_EXIST", "Address"=w461, "Port"=w460) -> (w462:T4)
            n253 = Enqueue Element(queue=w458, element=w462) -> ()  [unwired: 2 in, 3 out]
          }
          frame True {
            n254 = Bundle By Name(cluster=w474, "Data"="OK", "Address"=w473, "Port"=w472) -> (w476:T4)
            n255 = global read "ServerGlobalVariables.vi" "PlayerInfoMap"() -> (w465:T1)
            n256 = Enqueue Element(queue=w475, element=w476) -> ()  [unwired: 2 in, 3 out]
            n257 = in-place {
              in-place-border: w469 -> [w487]
              in-place-border: [w484] -> w471
              n258 = in-place-map #5(w465, w468) -> (w485:T7)  [unwired: 1 in, 1 out]
              n259 = Bundle By Name(cluster=w485, "Team"=w487) -> (w486:T7)
              n260 = Unbundle By Name(w485) -> ("Team"=w484:u8)
              n261 = in-place-map #5(w486, LVMapReplaceAction."Modify Entry only if found" ("action")) -> (w464:T1)  [unwired: 2 out]
            }
            n262 = call "LobbyBroadcaster.vi"("PlayerInfoMap"=w464) -> ()
            n263 = global read "ServerGlobalVariables.vi" "Teams"() -> (w466:set{u32}[])
            n264 = global write "ServerGlobalVariables.vi" "PlayerInfoMap"(w464) -> ()
            n265 = in-place {
              in-place-border: w468 -> [w482]
              n266 = in-place-array #6(w466, w471) -> (w483:set{u32})
              n267 = Remove From Set(10:w482, 11:w483) -> (3:w481:set{u32})  [unwired: 1 out]
              n268 = in-place-array #6(w481) -> (w470:set{u32}[])  [unwired: 1 out]
            }
            n269 = in-place {
              in-place-border: w468 -> [w479]
              n270 = in-place-array #7(w470, w469) -> (w480:set{u32})
              n271 = Insert Into Set(10:w479, 11:w480) -> (3:w478:set{u32})  [unwired: 1 out]
              n272 = in-place-array #7(w478) -> (w467:set{u32}[])  [unwired: 1 out]
            }
            n273 = global write "ServerGlobalVariables.vi" "Teams"(w467) -> ()
          }
        }
      }
    }
  }
  n274 = while {
    shift-right: [w492] -> _
    shift-left: T3."Wait Send Queue Ready" -> [w489]
    shift-right: [w491] -> _
    shift-left: T4 {"Data"="", "Address"=0, "Port"=0} -> [w490]
    stop <- FALSE stop-if-true
    # "Set Ready Handler"
    n275 = case shown="\"Process Data\"" w489 {
      tunnel: [w497 w501 T3."Process Data" T3."Poll Read Queue"] -> w492
      tunnel: [T4 {"Data"="", "Address"=0, "Port"=0} T4 {"Data"="", "Address"=0, "Port"=0} w507 T4 {"Data"="", "Address"=0, "Port"=0}] -> w491
      tunnel: w490 -> [_ _ _ w512]
      frame "Wait Send Queue Ready", Default {
        n276 = global read "ServerNetworkInterfaceGlobalVariables.vi" "Send Data Queue"() -> (w499:refnum<queue>)
        n277 = Get Queue Status(queue=w499) -> (error out=w498:errorcluster)  [unwired: 2 in, 7 out]
        n278 = Select(t=T3."Wait Send Queue Ready", s=w498, f=T3."Wait Receive Queue Ready") -> (s? t:f=w497:T3)
      }
      frame "Wait Receive Queue Ready" {
        n279 = global read "ServerNetworkInterfaceGlobalVariables.vi" "Receive Data Queue"() -> (w504:refnum<queue>)
        n280 = Get Queue Status(queue=w504) -> (error out=w505:errorcluster)  [unwired: 2 in, 7 out]
        n281 = Select(t=T3."Wait Receive Queue Ready", s=w505, f=T3."Poll Read Queue") -> (s? t:f=w501:T3)
      }
      frame "Poll Read Queue" {
        n282 = Obtain Queue(name (unnamed)="SET_READY", element data type=T4 {"Data"="", "Address"=0, "Port"=0}) -> (queue out=w508:refnum<queue>)  [unwired: 3 in, 2 out]
        n283 = Dequeue Element(queue=w508) -> (element=w507:T4)  [unwired: 2 in, 3 out]
      }
      frame "Process Data" {
        n284 = global read "ServerGlobalVariables.vi" "PlayerConnectionIDMap"() -> (w520:map{cluster{"Address":u32, "Port":u16}, u32})
        n285 = Unbundle By Name(w512) -> ("Data"=w523:string, "Address"=w516:u32, "Port"=w515:u16)
        n286 = Bundle("Address"=w516, "Port"=w515) -> (w519:cluster{"Address":u32, "Port":u16})  [unwired: 1 in]
        n287 = Look In Map(map=w520, key=w519) -> (key not found?=w517:bool, value=w514:u32)  [unwired: 1 in]
        n288 = Match True/False String(2:"FALSE" ("false string"), 3:"TRUE" ("true string"), 4:w523) -> (0:w513:bool)  [unwired: 1 out]
        n289 = Not(x=w517) -> (.not. x?=w518:bool)
        n290 = case shown="True" w518 {
          tunnel: w516 -> [w529 w540]
          tunnel: w515 -> [w528 w539]
          tunnel: w514 -> [_ w537]
          tunnel: w513 -> [_ w536]
          frame False {
            n291 = global read "ServerNetworkInterfaceGlobalVariables.vi" "Send Data Queue"() -> (w527:refnum<queue>)
            n292 = Bundle By Name(cluster=T4 {"Data"="", "Address"=0, "Port"=0}, "Data"="ERR_PLAYER_DOES_NOT_EXIST", "Address"=w529, "Port"=w528) -> (w526:T4)
            n293 = Enqueue Element(queue=w527, element=w526) -> ()  [unwired: 2 in, 3 out]
          }
          frame True {
            n294 = global read "ServerNetworkInterfaceGlobalVariables.vi" "Send Data Queue"() -> (w534:refnum<queue>)
            n295 = global read "ServerGlobalVariables.vi" "PlayerInfoMap"() -> (w535:T1)
            n296 = Bundle By Name(cluster=T4 {"Data"="", "Address"=0, "Port"=0}, "Data"="OK", "Address"=w540, "Port"=w539) -> (w532:T4)
            n297 = in-place {
              in-place-border: w536 -> [w541]
              n298 = in-place-map #8(w535, w537) -> (w542:T7)  [unwired: 1 in, 1 out]
              n299 = Bundle By Name(cluster=w542, "Ready"=w541) -> (w543:T7)
              n300 = in-place-map #8(w543, LVMapReplaceAction."Modify Entry only if found" ("action")) -> (w531:T1)  [unwired: 2 out]
            }
            n301 = Enqueue Element(queue=w534, element=w532) -> ()  [unwired: 2 in, 3 out]
            n302 = call "LobbyBroadcaster.vi"("PlayerInfoMap"=w531) -> ()
            n303 = global write "ServerGlobalVariables.vi" "PlayerInfoMap"(w531) -> ()
          }
        }
      }
    }
  }
  n304 = while {
    shift-right: [w548] -> _
    shift-left: T3."Wait Send Queue Ready" -> [w545]
    shift-right: [w547] -> _
    shift-left: T4 {"Data"="", "Address"=0, "Port"=0} -> [w546]
    stop <- FALSE stop-if-true
    # "Set Option Handler"
    n305 = case shown="\"Process Data\"" w545 {
      tunnel: [w553 w557 T3."Process Data" T3."Poll Read Queue"] -> w548
      tunnel: [T4 {"Data"="", "Address"=0, "Port"=0} T4 {"Data"="", "Address"=0, "Port"=0} w563 T4 {"Data"="", "Address"=0, "Port"=0}] -> w547
      tunnel: w546 -> [_ _ _ w570]
      frame "Wait Send Queue Ready", Default {
        n306 = global read "ServerNetworkInterfaceGlobalVariables.vi" "Send Data Queue"() -> (w555:refnum<queue>)
        n307 = Get Queue Status(queue=w555) -> (error out=w554:errorcluster)  [unwired: 2 in, 7 out]
        n308 = Select(t=T3."Wait Send Queue Ready", s=w554, f=T3."Wait Receive Queue Ready") -> (s? t:f=w553:T3)
      }
      frame "Wait Receive Queue Ready" {
        n309 = global read "ServerNetworkInterfaceGlobalVariables.vi" "Receive Data Queue"() -> (w560:refnum<queue>)
        n310 = Get Queue Status(queue=w560) -> (error out=w561:errorcluster)  [unwired: 2 in, 7 out]
        n311 = Select(t=T3."Wait Receive Queue Ready", s=w561, f=T3."Poll Read Queue") -> (s? t:f=w557:T3)
      }
      frame "Poll Read Queue" {
        n312 = Obtain Queue(name (unnamed)="SET_OPTION", element data type=T4 {"Data"="", "Address"=0, "Port"=0}) -> (queue out=w564:refnum<queue>)  [unwired: 3 in, 2 out]
        n313 = Dequeue Element(queue=w564) -> (element=w563:T4)  [unwired: 2 in, 3 out]
      }
      frame "Process Data" {
        n314 = global read "ServerGlobalVariables.vi" "PlayerConnectionIDMap"() -> (w581:map{cluster{"Address":u32, "Port":u16}, u32})
        n315 = Unbundle By Name(w570) -> ("Data"=w568:string, "Address"=w579:u32, "Port"=w578:u16)
        n316 = global read "ServerGlobalVariables.vi" "PlayerInfoMap"() -> (w576:T1)
        n317 = Bundle("Address"=w579, "Port"=w578) -> (w580:cluster{"Address":u32, "Port":u16})  [unwired: 1 in]
        n318 = Look In Map(map=w581, key=w580) -> (key not found?=w574:bool, value=w577:u32)  [unwired: 1 in]
        n319 = Look In Map(map=w576, key=w577) -> (value=w575:T7)  [unwired: 1 in, 1 out]
        n320 = Unbundle By Name(w575) -> ("Host"=w571:bool)
        n321 = Not(x=w574) -> (.not. x?=w572:bool)
        n322 = And(x=w572, y=w571) -> (x .and. y?=w573:bool)
        n323 = case shown="True" w573 {
          tunnel: w579 -> [w590 w602]
          tunnel: w578 -> [w589 w603]
          tunnel: w574 -> [w586 _]
          tunnel: w568 -> [_ w596]
          frame False {
            n324 = Select(t="ERR_PLAYER_DOES_NOT_EXIST" ("Data"), s=w586, f="ERR_PLAYER_IS_NOT_HOST") -> (s? t:f=w585:string)
            n325 = global read "ServerNetworkInterfaceGlobalVariables.vi" "Send Data Queue"() -> (w582:refnum<queue>)
            n326 = Bundle By Name(cluster=T4 {"Data"="", "Address"=0, "Port"=0}, "Data"=w585, "Address"=w590, "Port"=w589) -> (w584:T4)
            n327 = Enqueue Element(queue=w582, element=w584) -> ()  [unwired: 2 in, 3 out]
          }
          frame True {
            n328 = call <vilib>:"Delimited String to 1D String Array.vi"("delimiter"="|", "delimited string"=w596) -> ("string array"=w598:string[])  [unwired: 9 in]
            n329 = Array To Cluster(array=w598) -> (cluster=w599:T11)
            n330 = Unbundle(w599) -> ("string array[0]"=w594:string, "string array[1]"=w600:string)
            n331 = global read "ServerGlobalVariables.vi" "Options"() -> (w601:map{string, u32})
            n332 = Fract/Exp String To Number(string=w600) -> (number=w595:dbl)  [unwired: 3 in, 1 out]
            n333 = in-place {
              in-place-border: w595 -> [w618]
              n334 = in-place-map #9(w601, w594) -> ()  [unwired: 1 in, 2 out]
              n335 = in-place-map #9(w618, LVMapReplaceAction."Modify Entry only if found" ("action")) -> (w591:map{string, u32}, w605:bool)  [unwired: 1 out]
            }
            n336 = Not(x=w605) -> (.not. x?=w604:bool)
            n337 = Flatten To String(anything=w591) -> (data string=w592:string)  [unwired: 3 in, 2 out]
            n338 = global write "ServerGlobalVariables.vi" "Options"(w591) -> ()
            n339 = call "DataBroadcaster.vi"("Data"=w592, "Action"="OPTION_UPDATE") -> ()
            n340 = case shown="True" w604 {
              tunnel: w603 -> [w610 w616]
              tunnel: w602 -> [w609 w615]
              frame False {
                n341 = global read "ServerNetworkInterfaceGlobalVariables.vi" "Send Data Queue"() -> (w606:refnum<queue>)
                n342 = Bundle By Name(cluster=T4 {"Data"="", "Address"=0, "Port"=0}, "Data"="ERR_INVALID_OPTION", "Address"=w609, "Port"=w610) -> (w608:T4)
                n343 = Enqueue Element(queue=w606, element=w608) -> ()  [unwired: 2 in, 3 out]
              }
              frame True {
                n344 = global read "ServerNetworkInterfaceGlobalVariables.vi" "Send Data Queue"() -> (w612:refnum<queue>)
                n345 = Bundle By Name(cluster=T4 {"Data"="", "Address"=0, "Port"=0}, "Data"="OK", "Address"=w615, "Port"=w616) -> (w614:T4)
                n346 = Enqueue Element(queue=w612, element=w614) -> ()  [unwired: 2 in, 3 out]
              }
            }
          }
        }
      }
    }
  }
  n347 = while {
    shift-right: [w625] -> _
    shift-left: T5."Wait Send Queue Ready" -> [w622]
    shift-right: [w624] -> _
    shift-left: T4 {"Data"="", "Address"=0, "Port"=0} -> [w623]
    shift-right: [w621] -> _
    shift-left: u32 0 ("ID") -> [w620]
    stop <- FALSE stop-if-true
    # "Surrender Handler"
    n348 = case shown="\"Process Data\"" w622 {
      tunnel: [w631 w636 T5."Process Data" w653 w672] -> w625
      tunnel: [T4 {"Data"="", "Address"=0, "Port"=0} T4 {"Data"="", "Address"=0, "Port"=0} w643 T4 {"Data"="", "Address"=0, "Port"=0} T4 {"Data"="", "Address"=0, "Port"=0}] -> w624
      tunnel: w623 -> [_ _ _ w660 _]
      tunnel: [u32 0 ("ID") u32 0 ("ID") u32 0 ("ID") w652 w673] -> w621
      tunnel: w620 -> [_ _ _ _ w673]
      frame "Wait Send Queue Ready", Default {
        n349 = global read "ServerNetworkInterfaceGlobalVariables.vi" "Send Data Queue"() -> (w633:refnum<queue>)
        n350 = Get Queue Status(queue=w633) -> (error out=w632:errorcluster)  [unwired: 2 in, 7 out]
        n351 = Select(t=T5."Wait Send Queue Ready", s=w632, f=T5."Wait Receive Queue Ready") -> (s? t:f=w631:T5)
      }
      frame "Wait Receive Queue Ready" {
        n352 = global read "ServerNetworkInterfaceGlobalVariables.vi" "Receive Data Queue"() -> (w639:refnum<queue>)
        n353 = Get Queue Status(queue=w639) -> (error out=w640:errorcluster)  [unwired: 2 in, 7 out]
        n354 = Select(t=T5."Wait Receive Queue Ready", s=w640, f=T5."Poll Read Queue") -> (s? t:f=w636:T5)
      }
      frame "Poll Read Queue" {
        n355 = Obtain Queue(name (unnamed)="SURRENDER", element data type=T4 {"Data"="", "Address"=0, "Port"=0}) -> (queue out=w644:refnum<queue>)  [unwired: 3 in, 2 out]
        n356 = Dequeue Element(queue=w644) -> (element=w643:T4)  [unwired: 2 in, 3 out]
      }
      frame "Process Data" {
        n357 = Unbundle By Name(w660) -> ("Address"=w650:u32, "Port"=w649:u16)
        n358 = global read "ServerNetworkInterfaceGlobalVariables.vi" "Send Data Queue"() -> (w651:refnum<queue>)
        n359 = global read "ServerGlobalVariables.vi" "PlayerConnectionIDMap"() -> (w662:map{cluster{"Address":u32, "Port":u16}, u32})
        n360 = Bundle("OK", "Address"=w650, "Port"=w649) -> (w647:cluster{string, "Address":u32, "Port":u16})  [unwired: 1 in]
        n361 = global read "ServerGlobalVariables.vi" "PlayerInfoMap"() -> (w658:T1)
        n362 = Bundle("Address"=w650, "Port"=w649) -> (w661:cluster{"Address":u32, "Port":u16})  [unwired: 1 in]
        n363 = Enqueue Element At Opposite End(queue=w651, element=w647) -> ()  [unwired: 2 in, 3 out]
        n364 = Look In Map(map=w662, key=w661) -> (value=w652:u32)  [unwired: 1 in, 1 out]
        n365 = in-place {
          n366 = in-place-map #10(w658, w652) -> (w666:T7)  [unwired: 1 in, 1 out]
          n367 = Bundle By Name(cluster=w666, "Alive"=FALSE, "Lands"=set{cluster{"Row":u32, "Column":u32}} {}, "Army"=u32 0) -> (w667:T7)
          n368 = in-place-map #10(w667, LVMapReplaceAction."Modify Entry only if found" ("action")) -> (w657:T1)  [unwired: 2 out]
        }
        n369 = global write "ServerGlobalVariables.vi" "PlayerInfoMap"(w657) -> ()
        n370 = Empty Collection?(1:w657) -> (0:w656:bool)
        n371 = Select(t=T5."Process Data", s=w656, f=T5."Remove Land") -> (s? t:f=w653:T5)
      }
      frame "Remove Land" {
        n372 = global read "ServerGlobalVariables.vi" "PlayerInfoMap"() -> (w675:T1)
        n373 = in-place {
          in-place-border: [w677] -> w669
          n374 = in-place-map #11(w675, w673) -> (w687:T7)  [unwired: 1 in, 1 out]
          n375 = Unbundle By Name(w687) -> ("Lands"=w684:set{cluster{"Row":u32, "Column":u32}})
          n376 = Read Set Max & Min(11:w684) -> (1:w683:cluster{"Row":u32, "Column":u32})  [unwired: 1 out]
          n377 = global read "ServerGlobalVariables.vi" "FieldArray"() -> (w681:T9)
          n378 = Unbundle By Name(w683) -> ("Row"=w682:u32, "Column"=w680:u32)
          n379 = Remove From Set(10:w683, 11:w684) -> (3:w678:set{cluster{"Row":u32, "Column":u32}})  [unwired: 1 out]
          n380 = Bundle By Name(cluster=w687, "Lands"=w678) -> (w686:T7)
          n381 = in-place {
            n382 = in-place-array #12(w681, w682, w680) -> (w694:T10)
            n383 = Unbundle By Name(w694) -> ("City"=w692:bool, "General"=w691:bool)
            n384 = Or(x=w692, y=w691) -> (x .or. y?=w690:bool)
            n385 = Bundle By Name(cluster=w694, "Owner"=0, "City"=w690, "General"=FALSE) -> (w693:T10)
            n386 = in-place-array #12(w693) -> (w679:T9)  [unwired: 2 out]
          }
          n387 = Empty Collection?(1:w678) -> (0:w677:bool)
          n388 = global write "ServerGlobalVariables.vi" "FieldArray"(w679) -> ()
          n389 = in-place-map #11(w686, LVMapReplaceAction."Modify Entry only if found" ("action")) -> (w674:T1)  [unwired: 2 out]
        }
        n390 = global write "ServerGlobalVariables.vi" "PlayerInfoMap"(w674) -> ()
        n391 = Select(t=T5."Poll Read Queue", s=w669, f=T5."Remove Land") -> (s? t:f=w672:T5)
      }
    }
  }
  n392 = global write "ServerGlobalVariables.vi" "Options"(w21) -> ()
  n393 = global write "ServerGlobalVariables.vi" "PlayerColorArray"(u32[] [16711680, 2593535, 32768, 32896, 16419841, 15741670, 8388736, 10158337, 11775026, 10116644, 1061375, 5852325, 8759580, 16737896, 11829194, 11835761] ("PlayerColorArray")) -> ()
